vi "OAT Output Buffered Data (Even Angle, 1 Chan).vi"(0 "even-angle signal":cluster{"r0":dbl, "dr":dbl, "Y":dbl[]}={"r0"=0.0, "dr"=1.0, "Y"=[]} {"r0" format="%.2p"; "dr" format="%.2p"; "Y" format="%.2f"}, 2 "reset? (F)":bool, 7 "even-angle position info":T1, 11 "error in (no error)":errorcluster, 12 "buffer settings":T2) -> (4 "buffered even-angle signal":cluster{"r0":dbl, "dr":dbl, "Y":dbl[]}={"r0"=0.0, "dr"=1.0, "Y"=[]} {"r0" format="%.2p"; "dr" format="%.2p"; "Y" format="%.2f"}, 8 "buffered even-angle position info":T1, 15 "error out":errorcluster)   [LabVIEW 2017, in "SoundVib_OAUtility.lvlib"]
doc: "Buffers the input signals and returns them in first-in first-out (FIFO) mode. Use <B>buffer settings</B> to set the buffer size and units. Each instance of this VI maintains its own state; use the N Waveforms instance of this VI to process an array of channels. Wire data to the <B>XY signal</B> input to determine the polymorphic instance to use or manually select the instance."
uses:
  <vilib>/addons/Sound and Vibration/Order Analysis/Utility/SoundVib_OAUtility.lvlib
  <vilib>/addons/Sound and Vibration/Order Analysis/Misc/OAT Position Info.ctl
  <vilib>/addons/Sound and Vibration/Order Analysis/Utility/SubVIs/oa_Buffer Settings.ctl
  <vilib>/addons/_NISVFA/_Shared subVIs/Common/svc_Get Array Subset (Index).vi
  <vilib>/addons/_NISVFA/_Shared subVIs/Common/svc_Coerce Index and Length.vi
  <vilib>/addons/_NISVFA/_Shared subVIs/Common/svc_Conditional Merge Error.vi
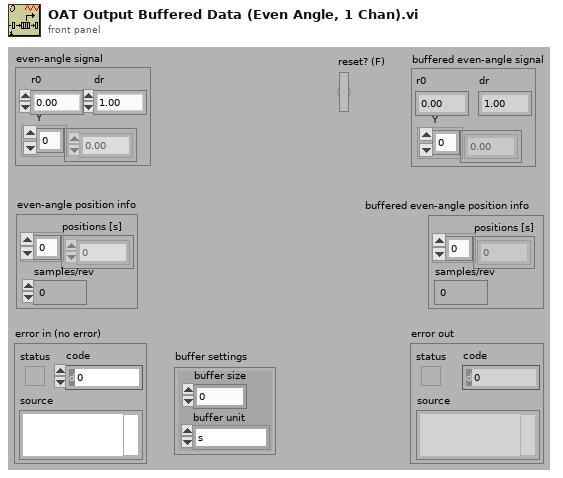
[diagram p1: front panel]
types:
  T1 = typedef "OAT Position Info.ctl" = cluster{"positions [s]":dbl[], "samples/rev":dbl}
  T2 = typedef "SoundVib_OAUtility.lvlib/oa_Buffer Settings.ctl" = cluster{"buffer size":dbl, "buffer unit":enum16{"s", "revolution", "# of samples"}}
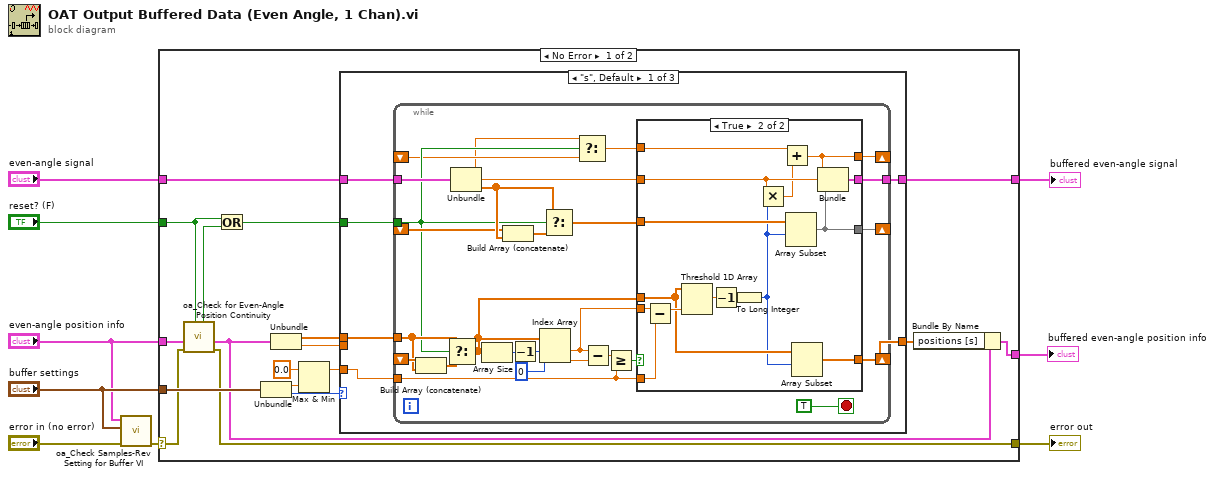
[diagram p0: block diagram]
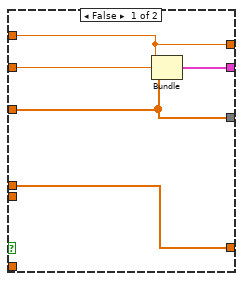
[diagram p2: hidden frame]
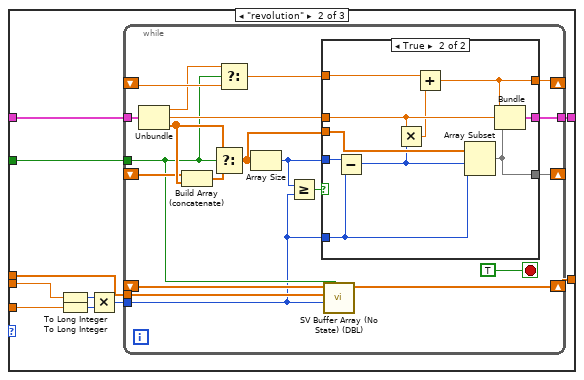
[diagram p3: hidden frame]
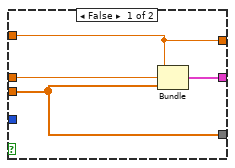
[diagram p4: hidden frame]
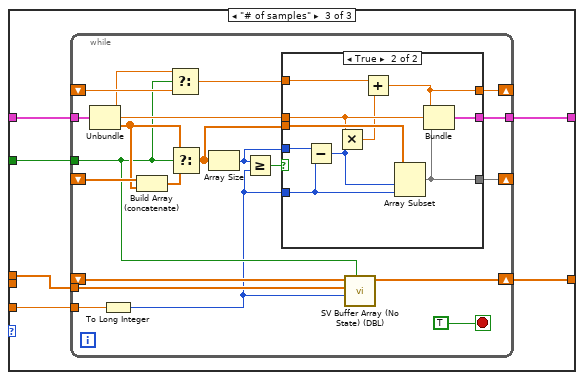
[diagram p5: hidden frame]
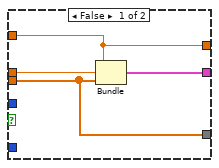
[diagram p6: hidden frame]
diagram:
  n1 = call <vilib>:"oa_Check Samples-Rev Setting for Buffer VI.vi"("error in (no error)"="error in (no error)", "buffer settings"="buffer settings", "position info"="even-angle position info") -> ("error out"=w5:errorcluster)  [unwired: 8 in]
  n2 = case shown="No Error" w5 {
    selector: w5 -> [w14 w166]
    tunnel: [w13 w166] -> w7
    tunnel: "buffer settings" -> [w27 _]
    tunnel: "even-angle signal" -> [w24 _]
    tunnel: "reset? (F)" -> [w17 _]
    tunnel: [w23 _] -> w6
    tunnel: "even-angle position info" -> [w20 _]
    tunnel: [w10 _] -> w1
    frame No Error {
      n3 = call <vilib>:"oa_Check for Even-Angle Position Continuity.vi"("reset in"=w17, "error in (no error)"=w14, "even-angle position info"=w20) -> ("error out"=w13:errorcluster, "even-angle position info dup"=w12:T1, "position not continuous"=w15:bool)  [unwired: 6 in]
      n4 = Or(x=w17, y=w15) -> (x .or. y?=w16:bool)
      n5 = Unbundle(w27) -> ("buffer size"=w21:dbl, "buffer unit"=w22:enum16{"s", "revolution", "# of samples"})
      n6 = Unbundle(w12) -> ("positions [s]"=w19:dbl[], "samples/rev"=w18:dbl)
      n7 = Max & Min(x=0.0, y=w21) -> (max(x,y)=w25:dbl)  [unwired: 1 out]
      n8 = case shown="\"s\", Default" w22 {
        tunnel: w25 -> [w32 w88 w128]
        tunnel: w24 -> [w30 w90 w130]
        tunnel: w16 -> [w29 w89 w129]
        tunnel: [w31 w87 w127] -> w23
        tunnel: w19 -> [w33 w86 w126]
        tunnel: w18 -> [_ w83 _]
        tunnel: [w28 w85 w125] -> w11
        frame "s", Default {
          n9 = while {
            tunnel: w33 -> [w42]
            tunnel: w32 -> [w51]
            tunnel: [w55] -> w31
            tunnel: w30 -> [w49]
            shift-right: [w54] -> _
            shift-left: _ -> [w46]
            tunnel: w29 -> [w39]
            shift-right: [w40] -> w28
            shift-left: _ -> [w43]
            shift-right: [w36] -> _
            shift-left: _ -> [w38]
            stop <- TRUE stop-if-true
            n10 = Build Array (concatenate)(w43, w42) -> (w41:dbl[])
            n11 = Select(t=w42, s=w39, f=w41) -> (s? t:f=w44:dbl[])
            n12 = Unbundle(w49) -> ("r0"=w34:dbl, "dr"=w45:dbl, "Y"=w47:dbl[])
            n13 = Array Size(array=w44) -> (size(s)=w60:i32)
            n14 = Build Array (concatenate)(w46, w47) -> (w50:dbl[])
            n15 = Decrement(x=w60) -> (x-1=w59:i32)
            n16 = Index Array(array=w44, index #1=w59, index #2=0 ("index")) -> (element #1=w52:dbl, element #2=w35:dbl)
            n17 = Select(t=w47, s=w39, f=w50) -> (s? t:f=w48:dbl[])
            n18 = Select(t=w34, s=w39, f=w38) -> (s? t:f=w37:dbl)
            n19 = Subtract(x=w52, y=w35) -> (x-y=w57:dbl)
            n20 = Greater Or Equal?(x=w57, y=w51) -> (x >= y?=w56:bool)
            n21 = case shown="True" w56 {
              tunnel: [w65 w75] -> w55
              tunnel: [w64 w73] -> w54
              tunnel: w44 -> [w62 w71]
              tunnel: w52 -> [_ w80]
              tunnel: w51 -> [_ w79]
              tunnel: w48 -> [w64 w74]
              tunnel: w45 -> [w63 w69]
              tunnel: w37 -> [w61 w68]
              tunnel: [w62 w72] -> w40
              tunnel: [w61 w66] -> w36
              frame False {
                n22 = Bundle("r0"=w61, "dr"=w63, "Y"=w64) -> (w65:cluster{"r0":dbl, "dr":dbl, "Y":dbl[]})  [unwired: 1 in]
              }
              frame True {
                n23 = Subtract(x=w80, y=w79) -> (x-y=w78:dbl)
                n24 = Threshold 1D Array(2:w78, 3:w71) -> (0:w77:dbl)  [unwired: 1 in]
                n25 = Decrement(x=w77) -> (x-1=w76:dbl)
                n26 = To Long Integer(number=w76) -> (32bit integer=w70:i32)
                n27 = Multiply(x=w69, y=w70) -> (x*y=w67:dbl)
                n28 = Add(x=w68, y=w67) -> (x+y=w66:dbl)
                n29 = Array Subset(array=w74, index=w70) -> (w73:dbl[])  [unwired: 1 in]
                n30 = Array Subset(array=w71, index=w70) -> (w72:dbl[])  [unwired: 1 in]
                n31 = Bundle(w66, "dr"=w69, w73) -> (w75:cluster{dbl, "dr":dbl, dbl[]})  [unwired: 1 in]
              }
            }
          }
        }
        frame "revolution" {
          n32 = To Long Integer(number=w83) -> (32bit integer=w84:i32)
          n33 = To Long Integer(number=w88) -> (32bit integer=w82:i32)
          n34 = Multiply(x=w84, y=w82) -> (x*y=w81:i32)
          n35 = while {
            tunnel: w90 -> [w110]
            shift-right: [w107] -> _
            shift-left: _ -> [w102]
            tunnel: w89 -> [w92]
            tunnel: [w106] -> w87
            shift-right: [w96] -> _
            shift-left: _ -> [w99]
            shift-right: [w95] -> w85
            shift-left: _ -> [w94]
            tunnel: w86 -> [w93]
            tunnel: w81 -> [w91]
            stop <- TRUE stop-if-true
            n36 = Unbundle(w110) -> ("r0"=w98:dbl, "dr"=w101:dbl, "Y"=w103:dbl[])
            n37 = Build Array (concatenate)(w102, w103) -> (w104:dbl[])
            n38 = Select(t=w103, s=w92, f=w104) -> (s? t:f=w108:dbl[])
            n39 = Select(t=w98, s=w92, f=w99) -> (s? t:f=w97:dbl)
            n40 = Array Size(array=w108) -> (size(s)=w100:i32)
            n41 = Greater Or Equal?(x=w100, y=w91) -> (x >= y?=w105:bool)
            n42 = case shown="True" w105 {
              tunnel: w108 -> [w112 w124]
              tunnel: w100 -> [_ w122]
              tunnel: [w112 w120] -> w107
              tunnel: [w114 w123] -> w106
              tunnel: w91 -> [_ w121]
              tunnel: w101 -> [w113 w118]
              tunnel: w97 -> [w111 w117]
              tunnel: [w111 w115] -> w96
              frame False {
                n43 = Bundle("r0"=w111, "dr"=w113, "Y"=w112) -> (w114:cluster{"r0":dbl, "dr":dbl, "Y":dbl[]})  [unwired: 1 in]
              }
              frame True {
                n44 = Subtract(x=w122, y=w121) -> (x-y=w119:i32)
                n45 = Multiply(x=w118, y=w119) -> (x*y=w116:dbl)
                n46 = Add(x=w117, y=w116) -> (x+y=w115:dbl)
                n47 = Array Subset(array=w124, index=w119, length=w121) -> (w120:dbl[])
                n48 = Bundle(w115, "dr"=w118, w120) -> (w123:cluster{dbl, "dr":dbl, dbl[]})  [unwired: 1 in]
              }
            }
            n49 = call <vilib>:"SV Buffer Array (No State) (DBL).vi"("clear buffer (False)"=w92, "buffer length  [samples] (-1 = unlimited)"=w91, "Y"=w93, "buffer in"=w94) -> ("buffer out"=w95:dbl[])  [unwired: 7 in]
          }
        }
        frame "# of samples" {
          n50 = while {
            tunnel: w130 -> [w151]
            shift-right: [w147] -> _
            shift-left: _ -> [w144]
            tunnel: w129 -> [w133]
            tunnel: w128 -> [w149]
            tunnel: [w146] -> w127
            shift-right: [w136] -> _
            shift-left: _ -> [w139]
            shift-right: [w134] -> w125
            shift-left: _ -> [w135]
            tunnel: w126 -> [w132]
            stop <- TRUE stop-if-true
            n51 = Unbundle(w151) -> ("r0"=w138:dbl, "dr"=w141:dbl, "Y"=w142:dbl[])
            n52 = To Long Integer(number=w149) -> (32bit integer=w131:i32)
            n53 = Build Array (concatenate)(w144, w142) -> (w143:dbl[])
            n54 = Select(t=w138, s=w133, f=w139) -> (s? t:f=w137:dbl)
            n55 = Select(t=w142, s=w133, f=w143) -> (s? t:f=w140:dbl[])
            n56 = Array Size(array=w140) -> (size(s)=w148:i32)
            n57 = Greater Or Equal?(x=w148, y=w131) -> (x >= y?=w145:bool)
            n58 = case shown="True" w145 {
              tunnel: w140 -> [w155 w163]
              tunnel: w131 -> [_ w164]
              tunnel: w148 -> [_ w165]
              tunnel: [w155 w162] -> w147
              tunnel: [w154 w161] -> w146
              tunnel: w141 -> [w153 w159]
              tunnel: w137 -> [w152 w158]
              tunnel: [w152 w156] -> w136
              frame False {
                n59 = Bundle("r0"=w152, "dr"=w153, "Y"=w155) -> (w154:cluster{"r0":dbl, "dr":dbl, "Y":dbl[]})  [unwired: 1 in]
              }
              frame True {
                n60 = Subtract(x=w165, y=w164) -> (x-y=w160:i32)
                n61 = Multiply(x=w159, y=w160) -> (x*y=w157:dbl)
                n62 = Add(x=w158, y=w157) -> (x+y=w156:dbl)
                n63 = Array Subset(array=w163, index=w160, length=w164) -> (w162:dbl[])
                n64 = Bundle(w156, "dr"=w159, w162) -> (w161:cluster{dbl, "dr":dbl, dbl[]})  [unwired: 1 in]
              }
            }
            n65 = call <vilib>:"SV Buffer Array (No State) (DBL).vi"("clear buffer (False)"=w133, "buffer length  [samples] (-1 = unlimited)"=w131, "Y"=w132, "buffer in"=w135) -> ("buffer out"=w134:dbl[])  [unwired: 7 in]
          }
        }
      }
      n66 = Bundle By Name(cluster=w12, "positions [s]"=w11) -> (w10:T1)
    }
    frame Error {
    }
  }
  "error out" <- w7
  "buffered even-angle signal" <- w6
  "buffered even-angle position info" <- w1
